vi "Read_Wrap_Simple.vi"() -> (1 "Value":T1)   [LabVIEW 2021, in "Var_Bool.lvclass"]
uses:
  Var_Bool.lvclass
  Var_Bool.lvclass/Var_Bool.ctl
  Type.ctl
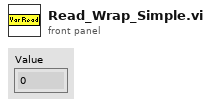
[diagram p1: front panel]
types:
  T1 = typedef "Var_Bool.lvclass/Type.ctl" = dbl
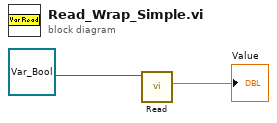
[diagram p0: block diagram]
diagram:
  n1 = call-dynamic "Read.vi"("Numeric in"=refnum<class "Var_Bool.lvclass"> refnum ("Constants.lvlib:Numeric.lvclass")) -> ("Numeric"=→"Value":T1)  [unwired: 8 in, 2 out]
